vi "Versionshistorie.vi"(11 "Abfrage":bool) -> (2 "v-PC":string, 3 "v-cRIO":string, 5 "Projekt":string)   [LabVIEW 2020]
uses:
  <vilib>/Utility/Data Type/NI_Data Type.lvlib
  Allgemein/allgemeine Sub-VIs.lvlib
panel:
  out "PC":i32
  out "cRIO":i32
  in  "Ebene":enum16{"cRIO", "PC"}(ring)=enum."PC"
  out "Element":string
  in  "Version":string
  in  "Version manuell vorgeben":bool
  in  "Baumstruktur":string(tree)
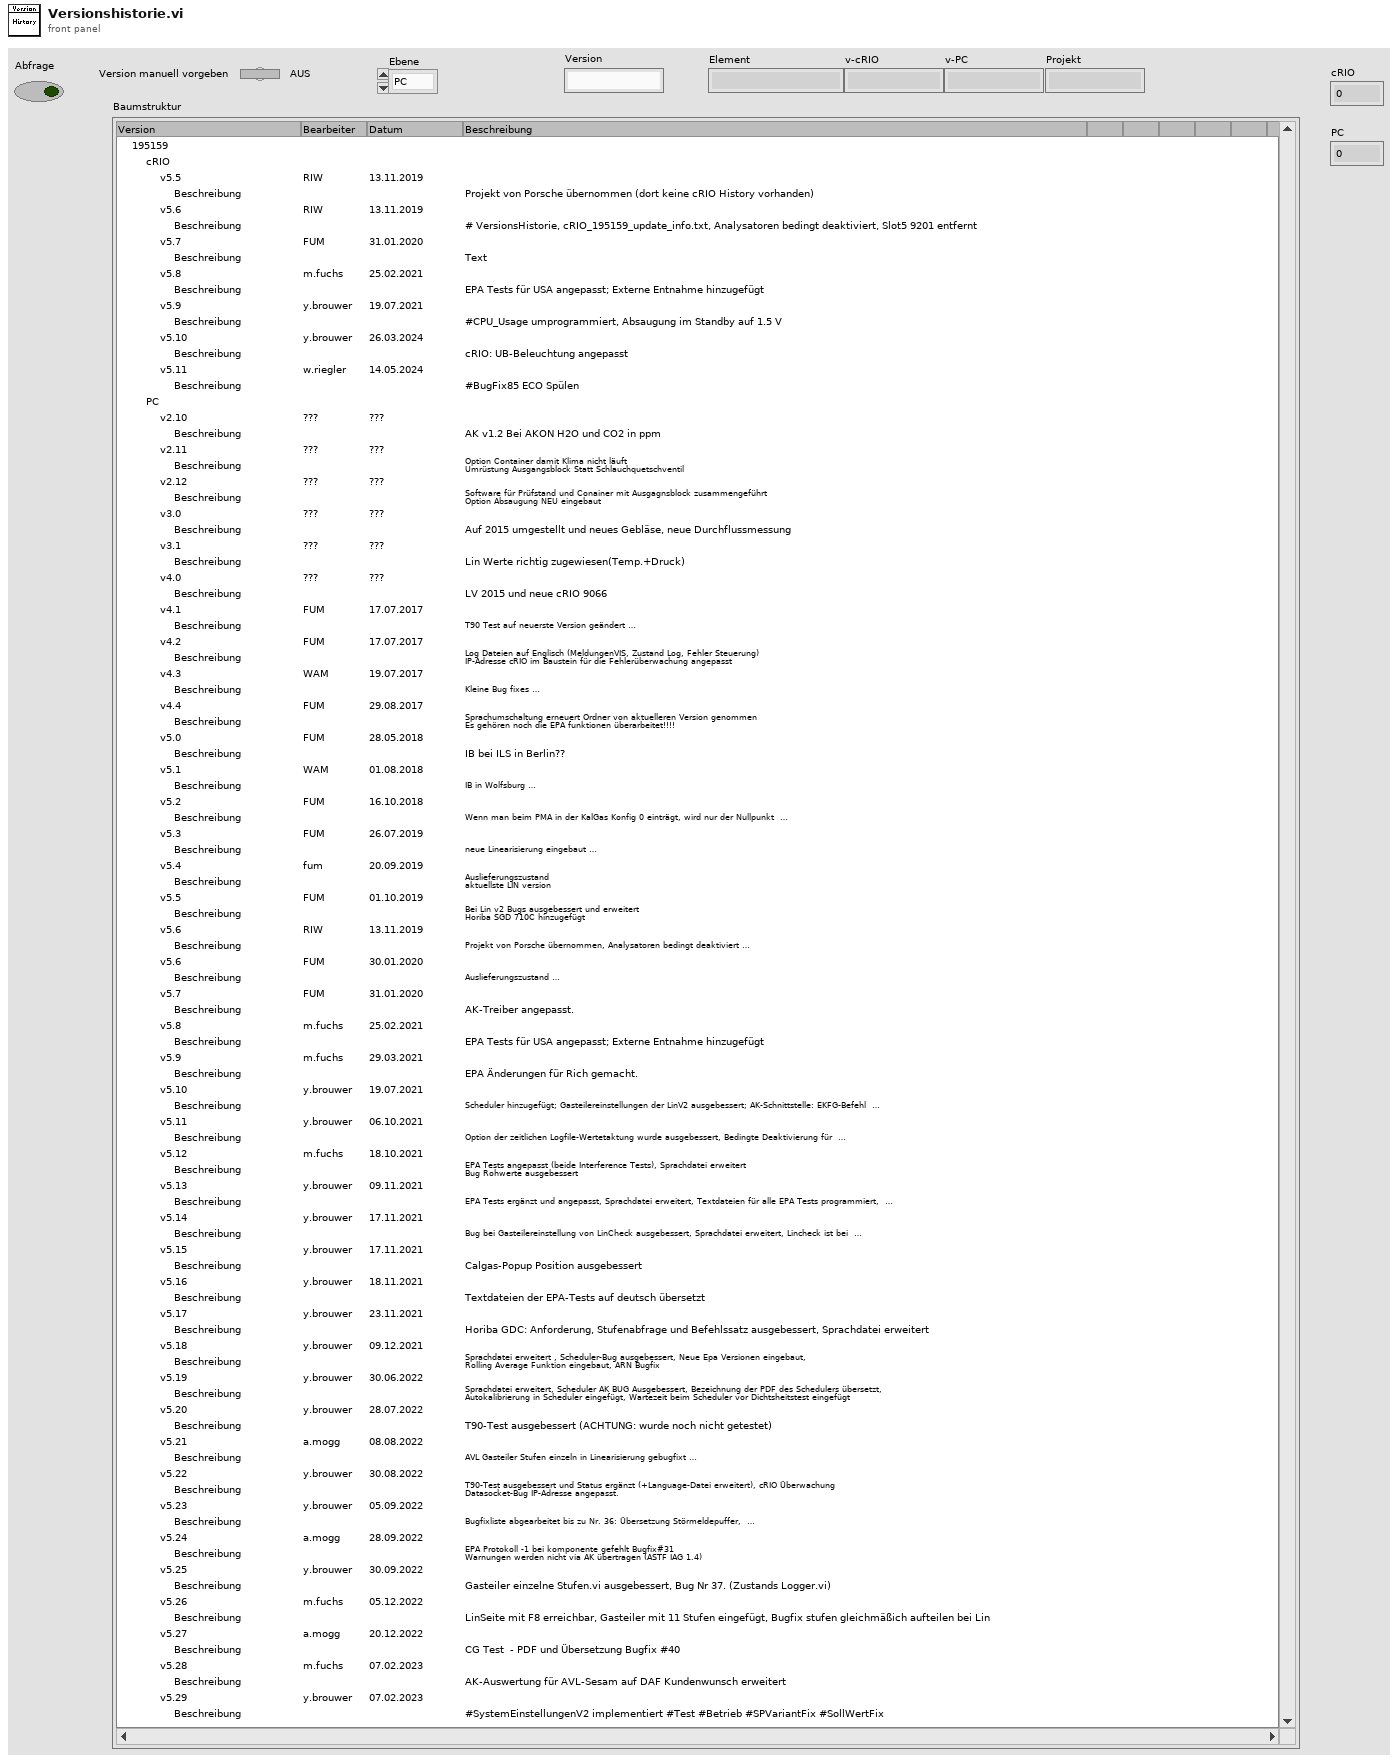
[diagram p1: front panel]
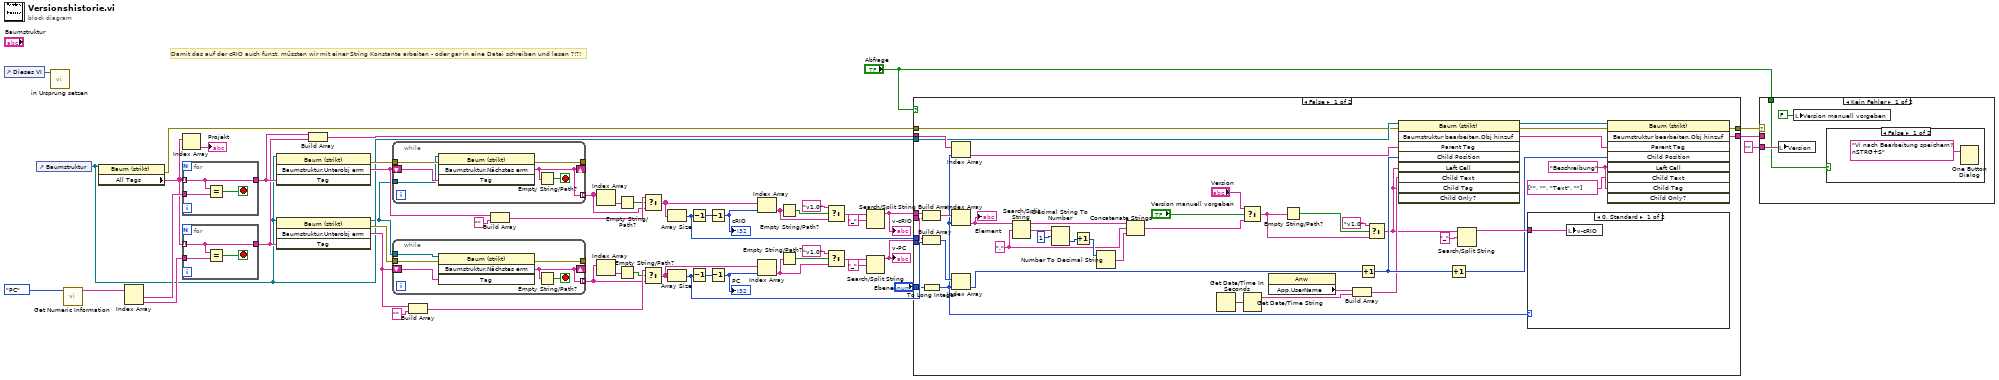
[diagram p0: block diagram]
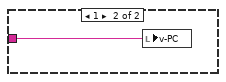
[diagram p2: hidden frame]
diagram:
  # "Damit das auf der cRIO auch funzt, müssten wir mit einer String Konstante arbeiten - oder gar in eine Datei schreiben und lesen ?!?!"
  n1 = control-ref of="Dieses VI"() -> (w8:refnum<vi>)
  n2 = control-ref of="Baumstruktur"() -> (w6:refnum<vi>)
  n3 = call "in Ursprung setzen.vi"("VI Referenz"=w8) -> ()  [unwired: 10 in, 1 out]
  n4 = call <vilib>:"Get Numeric Information.vi"("variant"=enum16{"cRIO", "PC"}."PC" ("Ebene")) -> ("enum names"=w49:string[])  [unwired: 7 in, 3 out]
  n5 = property class="Baum (strikt)"(reference=w6) -> (error out=w5:errorcluster, "All Tags"=w7:string[])  [unwired: 1 in, 1 out]
  n6 = Index Array(array=w49) -> (element #1=w48:string, element #2=w47:string)  [unwired: 2 in]
  n7 = Index Array(array=w7) -> (element=→"Projekt":string)  [unwired: 1 in]
  n8 = for {
    tunnel: w7 -> [w53] mode=indexing
    tunnel: w48 -> [w55]
    tunnel: [w53] -> w43
    stop <- w54 stop-if-true
    n9 = Equal?(x=w53, y=w55) -> (x = y?=w54:bool)
  }
  n10 = for {
    tunnel: w7 -> [w56] mode=indexing
    tunnel: w47 -> [w58]
    tunnel: [w56] -> w42
    stop <- w57 stop-if-true
    n11 = Equal?(x=w56, y=w58) -> (x = y?=w57:bool)
  }
  n12 = invoke on="Methodenknoten" class="Baum (strikt)" method="Baumstruktur.Unterobj erm"(reference=w6, "Tag"=w43) -> (error out=w51:errorcluster, "Navigate Tree:Get Child"=w29:string)  [unwired: 2 in, 2 out]
  n13 = invoke on="Methodenknoten" class="Baum (strikt)" method="Baumstruktur.Unterobj erm"(reference=w6, "Tag"=w42) -> (reference out=w2:refnum<vi>, error out=w44:errorcluster, "Navigate Tree:Get Child"=w25:string)  [unwired: 2 in, 1 out]
  n14 = Build Array(w43, w42) -> (w45:string[])
  n15 = while {
    tunnel: w51 -> [w63]
    tunnel: [w60] -> _
    shift-right: [w61] -> _
    shift-left: w29 -> [w62]
    tunnel: [w61] -> w21 mode=indexing
    tunnel: w2 -> [w59]
    stop <- w64 stop-if-true
    n16 = invoke on="Methodenknoten" class="Baum (strikt)" method="Baumstruktur.Nächstes erm"(reference=w59, error in=w63, "Tag"=w62) -> (error out=w60:errorcluster, "Navigate Tree:Get Next Item"=w61:string)  [unwired: 1 in, 2 out]
    n17 = Empty String/Path?(string/path=w61) -> (empty?=w64:bool)
  }
  n18 = while {
    tunnel: w44 -> [w69]
    tunnel: [w68] -> _
    shift-right: [w66] -> _
    shift-left: w25 -> [w67]
    tunnel: [w66] -> w18 mode=indexing
    tunnel: w2 -> [w65]
    stop <- w70 stop-if-true
    n19 = invoke on="Methodenknoten" class="Baum (strikt)" method="Baumstruktur.Nächstes erm"(reference=w65, error in=w69, "Tag"=w67) -> (error out=w68:errorcluster, "Navigate Tree:Get Next Item"=w66:string)  [unwired: 1 in, 2 out]
    n20 = Empty String/Path?(string/path=w66) -> (empty?=w70:bool)
  }
  n21 = Build Array(w25, "" ("Element")) -> (w26:string[])
  n22 = Build Array(w29, "" ("Element")) -> (w28:string[])
  n23 = Index Array(array=w21) -> (element=w20:string)  [unwired: 1 in]
  n24 = Index Array(array=w18) -> (element=w17:string)  [unwired: 1 in]
  n25 = Empty String/Path?(string/path=w20) -> (empty?=w19:bool)
  n26 = Empty String/Path?(string/path=w17) -> (empty?=w16:bool)
  n27 = Select(t=w28, s=w19, f=w21) -> (s? t:f=w27:string[])
  n28 = Select(t=w26, s=w16, f=w18) -> (s? t:f=w24:string[])
  n29 = Array Size(array=w27) -> (size(s)=w40:i32)
  n30 = Array Size(array=w24) -> (size(s)=w41:i32)
  n31 = Decrement(x=w40) -> (x-1=w36:i32)
  n32 = Decrement(x=w41) -> (x-1=w37:i32)
  n33 = Decrement(x=w36) -> (x-1=w39:i32)
  "cRIO" <- w39
  n34 = Decrement(x=w37) -> (x-1=w38:i32)
  "PC" <- w38
  n35 = Index Array(array=w27, index=w39) -> (element=w30:string)
  n36 = Index Array(array=w24, index=w38) -> (element=w31:string)
  n37 = Empty String/Path?(string/path=w30) -> (empty?=w35:bool)
  n38 = Empty String/Path?(string/path=w31) -> (empty?=w33:bool)
  n39 = Select(t="v1.0", s=w35, f=w30) -> (s? t:f=w14:string)
  n40 = Select(t="v1.0", s=w33, f=w31) -> (s? t:f=w11:string)
  n41 = Search/Split String(string=w14, search string/char (-)="_" ("Regulärer Ausdruck")) -> (substring before match=w13:string)  [unwired: 1 in, 2 out]
  "v-cRIO" <- w13
  n42 = Search/Split String(string=w11, search string/char (-)="_" ("Regulärer Ausdruck")) -> (substring before match=w10:string)  [unwired: 1 in, 2 out]
  "v-PC" <- w10
  n43 = case shown="False" "Abfrage" {
    tunnel: "Ebene" -> [w100 _]
    tunnel: w45 -> [w99 _]
    tunnel: w41 -> [w95 _]
    tunnel: w40 -> [w94 _]
    tunnel: w13 -> [w87 _]
    tunnel: w10 -> [w86 _]
    tunnel: w6 -> [w84 _]
    tunnel: w5 -> [w83 w116]
    tunnel: [w72 w116] -> w4
    tunnel: [w71 _] -> w3
    frame False {
      w74 = "Beschreibung" ("Linker Zellen-String")
      w107 = "." ("Regulärer Ausdruck")
      n44 = Build Array(w87, w86) -> (w98:string[])
      n45 = Build Array(w94, w95) -> (w97:i32[])
      n46 = To Long Integer(number=w100) -> (32bit integer=w90:i32)
      n47 = Index Array(array=w99, index=w90) -> (element=w82:string)
      n48 = Index Array(array=w98, index=w90) -> (element=w85:string)
      "Element" <- w85
      n49 = Index Array(array=w97, index=w90) -> (element=w96:i32)
      n50 = Search/Split String(string=w85, search string/char (-)=w107) -> (substring before match=w108:string, match + rest of string=w111:string)  [unwired: 1 in, 1 out]
      n51 = Decimal String To Number(string=w111, offset=1 ("Offset")) -> (number=w110:i32)  [unwired: 1 in, 1 out]
      n52 = Increment(x=w110) -> (x+1=w109:i32)
      n53 = Number To Decimal String(number=w109) -> (decimal integer string=w106:string)  [unwired: 1 in]
      n54 = Concatenate Strings(w108, w107, w106) -> (w103:string)
      n55 = Get Date/Time In Seconds() -> (seconds since 1Jan1904=w113:timestamp)
      n56 = Select(t="Version", s="Version manuell vorgeben", f=w103) -> (s? t:f=w92:string)
      n57 = Get Date/Time String(seconds (now)=w113) -> (date string=w101:string)  [unwired: 2 in, 1 out]
      n58 = property class="Anw"() -> ("App.UserName"=w102:string)  [unwired: 2 in, 2 out]
      n59 = Empty String/Path?(string/path=w92) -> (empty?=w93:bool)
      n60 = Build Array(w102, w101) -> (w80:string[])
      n61 = Increment(x=w96) -> (x+1=w81:i32)
      n62 = Select(t="v1.0", s=w93, f=w92) -> (s? t:f=w79:string)
      n63 = invoke on="Methodenknoten" class="Baum (strikt)" method="Baumstruktur bearbeiten.Obj hinzuf"(reference=w84, error in=w83, "Parent Tag"=w82, "Child Position"=w81, "Left Cell"=w79, "Child Text"=w80, "Child Tag"=w79) -> (reference out=w76:refnum<vi>, error out=w78:errorcluster, "Edit Tree Items:Add Item"=w77:string)  [unwired: 2 in, 6 out]
      n64 = Increment(x=w81) -> (x+1=w75:i32)
      n65 = Search/Split String(string=w79, search string/char (-)="_" ("Regulärer Ausdruck")) -> (substring before match=w88:string)  [unwired: 1 in, 2 out]
      n66 = case shown="0, Standard" w90 {
        tunnel: w88 -> [w114 w115]
        frame 0, Default {
          n67 = local write "v-cRIO"(w114) -> ()
        }
        frame 1 {
          n68 = local write "v-PC"(w115) -> ()
        }
      }
      n69 = invoke on="Methodenknoten" class="Baum (strikt)" method="Baumstruktur bearbeiten.Obj hinzuf"(reference=w76, error in=w78, "Parent Tag"=w77, "Child Position"=w75, "Left Cell"=w74, "Child Text"=string[] ["", "", "Text", ""] ("Unterobjekttext"), "Child Tag"=w74) -> (error out=w72:errorcluster, "Edit Tree Items:Add Item"=w71:string)  [unwired: 2 in, 7 out]
    }
    frame True {
    }
  }
  n70 = case shown="Kein Fehler" w4 {
    tunnel: "" ("Version") -> [w119 _]
    tunnel: w3 -> [_ _]
    tunnel: "Abfrage" -> [w117 _]
    frame No Error {
      n71 = local write "Version"(w119) -> ()
      n72 = local write "Version manuell vorgeben"(FALSE ("Version vorgeben")) -> ()
      n73 = case shown="False" w117 {
        frame False {
          n74 = One Button Dialog(message="Vi nach Bearbeitung speichern!\nSTRG+S" ("Nachricht")) -> ()  [unwired: 1 in, 1 out]
        }
        frame True {
        }
      }
    }
    frame Error {
    }
  }
